vi "PCO_GetRecordingStruct.vi"(8 "error in (no error)":errorcluster {"code" format="%x"}, 11 "ph":u64) -> (0 "error out":errorcluster {"code" format="%x"}, 1 "strRecording":T1, 2 "ErrorMessage":i32 format="%x", 3 "ph out":u64)   [LabVIEW 2019, in "SDK.lvlib" / "RecordingControl.lvlib"]
doc: "<b>Description:</b>\nRecording control information is queried from the camera and the variables of the PCO_Recording structure are filled with this information. This function is a combined version of the functions, which request information about the recording control related parameter. For a detailed description of each parameter see the functions in this chapter.\n\n<b>Supported camera type:</b>\nAll cameras\n\n<b>Descriptor dependency:</b>\nNone"
uses:
  RecordingControl.lvlib
  Structures/Structures.lvlib
  <vilib>/Utility/miscctls.llb/LVDateTimeRec.ctl
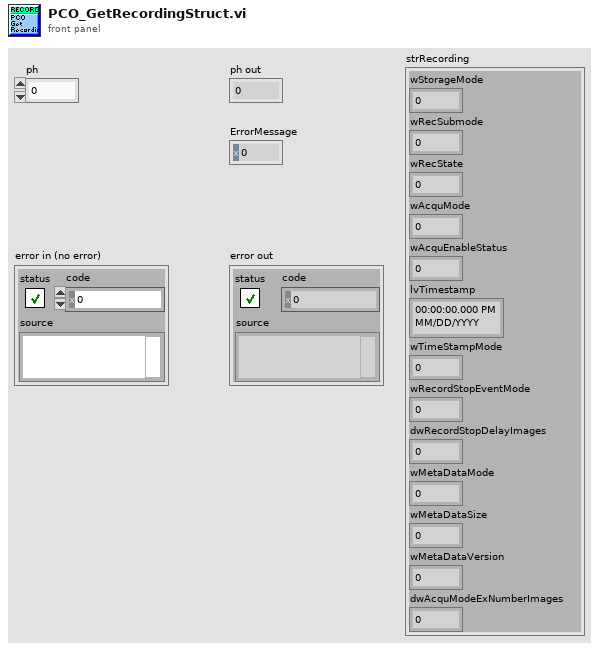
[diagram p1: front panel]
types:
  T1 = cluster{"wStorageMode":u16, "wRecSubmode":u16, "wRecState":u16, "wAcquMode":u16, "wAcquEnableStatus":u16, "lvTimestamp":timestamp, "wTimeStampMode":u16, "wRecordStopEventMode":u16, "dwRecordStopDelayImages":u32, "wMetaDataMode":u16, "wMetaDataSize":u16, "wMetaDataVersion":u16, "dwAcquModeExNumberImages":u32}
  T2 = typedef "LVDateTimeRec.ctl" = cluster{"fractional second":dbl, "second":i32, "minute":i32, "hour":i32, "day of month":i32, "month":i32, "year":i32, "day of week":i32, "day of year":i32, "DST":i32}
  T3 = cluster{"wSize":u16, "wStorageMode":u16, "wRecSubmode":u16, "wRecState":u16, "wAcquMode":u16, "wAcquEnableStatus":u16, "ucDay":u8, "ucMonth":u8, "wYear":u16, "wHour":u16, "ucMin":u8, "ucSec":u8, "wTimeStampMode":u16, "wRecordStopEventMode":u16, "dwRecordStopDelayImages":u32, "wMetaDataMode":u16, "wMetaDataSize":u16, "wMetaDataVersion":u16, "ZZwDummy1":u16, "dwAcquModeExNumberImages":u32, "dwAcquModeExReserved":cluster{u32, u32, u32, u32}, "ZZwDummy":cluster{u16, u16, u16, u16, u16, u16, u16, u16, u16, u16, u16, u16, u16, u16, u16, u16, u16, u16, u16, u16, u16, u16}}
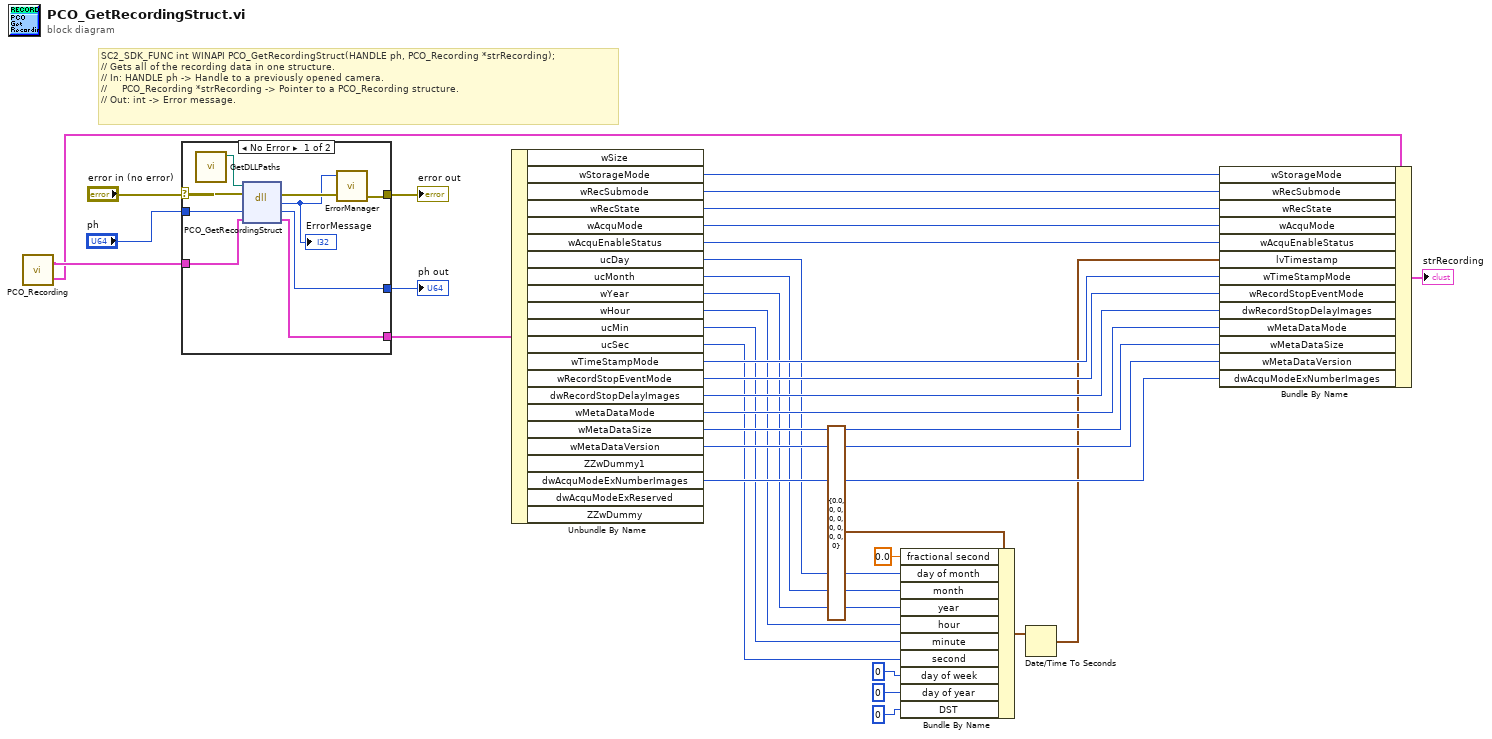
[diagram p0: block diagram]
diagram:
  # "SC2_SDK_FUNC int WINAPI PCO_GetRecordingStruct(HANDLE ph, PCO_Recording *strRecording);\n// Gets all of the recording data in one structure.\n// In: HANDLE ph -> Handle to a previously opened camera.\n//     PCO_Recording *strRecording -> Pointer to a PCO_Recording structure.\n// Out: int -> Error message."
  n1 = call "PCO_Recording.vi"() -> ("PCO_Recording"=w27:T1, "PCO_Recording_Raw"=w29:T3)  [unwired: 4 in, 2 out]
  n2 = case shown="No Error" "error in (no error)" {
    selector: "error in (no error)" -> [w38 w45]
    tunnel: "ph" -> [w42 w44]
    tunnel: [w41 w44] -> w32
    tunnel: w29 -> [w40 w43]
    tunnel: [w39 w43] -> w28
    tunnel: [w36 w45] -> w31
    frame No Error {
      n3 = call "GetDLLPaths.vi"() -> ("SC2_Cam_Path"=w34:path)  [unwired: 9 in, 2 out]
      n4 = dll-call lib="?" fn="PCO_GetRecordingStruct"(path in=w34, error in=w38, "ph"=w42, "strRecording"=w40) -> (error out=w37:errorcluster, "return type"=w35:i32, "ph"=w41:u64, "strRecording"=w39:T3)  [unwired: 1 in, 1 out]
      "ErrorMessage" <- w35
      n5 = call "ErrorManager.vi"("error in (no error)"=w37, "error code"=w35) -> ("error out"=w36:errorcluster)  [unwired: 3 in]
    }
    frame Error {
    }
  }
  "ph out" <- w32
  "error out" <- w31
  n6 = Unbundle By Name(w28) -> ("wStorageMode"=w26:u16, "wRecSubmode"=w25:u16, "wRecState"=w24:u16, "wAcquMode"=w23:u16, "wAcquEnableStatus"=w22:u16, "ucDay"=w6:u8, "ucMonth"=w5:u8, "wYear"=w4:u16, "wHour"=w3:u16, "ucMin"=w2:u8, "ucSec"=w1:u8, "wTimeStampMode"=w21:u16, "wRecordStopEventMode"=w20:u16, "dwRecordStopDelayImages"=w19:u32, "wMetaDataMode"=w18:u16, "wMetaDataSize"=w17:u16, "wMetaDataVersion"=w16:u16, "dwAcquModeExNumberImages"=w15:u32)  [unwired: 4 out]
  n7 = Bundle By Name(cluster=T2 {"fractional second"=0.0, "second"=0, "minute"=0, "hour"=0, "day of month"=0, "month"=0, "year"=0, "day of week"=0, "day of year"=0, "DST"=0} ("date time rec"), "fractional second"=0.0, "day of month"=w6, "month"=w5, "year"=w4, "hour"=w3, "minute"=w2, "second"=w1, "day of week"=0, "day of year"=0, "DST"=0) -> (w14:T2)
  n8 = Date/Time To Seconds(2:w14) -> (0:w9:timestamp)  [unwired: 1 in]
  n9 = Bundle By Name(cluster=w27, "wStorageMode"=w26, "wRecSubmode"=w25, "wRecState"=w24, "wAcquMode"=w23, "wAcquEnableStatus"=w22, "lvTimestamp"=w9, "wTimeStampMode"=w21, "wRecordStopEventMode"=w20, "dwRecordStopDelayImages"=w19, "wMetaDataMode"=w18, "wMetaDataSize"=w17, "wMetaDataVersion"=w16, "dwAcquModeExNumberImages"=w15) -> (→"strRecording":T1)
